vi "O to G v1.vi"(8 "height":dbl[](array[numeric]) format="%#_9g", 9 "south chip":dbl[](array[numeric]) format="%#_9g", 10 "north chip":dbl[](array[numeric]) format="%#_9g", 11 "Input file":path) -> (1 "output BR":dbl[](array[numeric]), 2 "output BL":dbl[](array[numeric]), 3 "output TL":dbl[](array[numeric]))   [LabVIEW 2016]
uses:
  <vilib>/Analysis/coordinate.llb/2D Cartesian Coordinate Rotation (Scalar).vi
  <vilib>/Utility/file.llb/Read Delimited Spreadsheet (DBL).vi
  <vilib>/Analysis/NI_AALPro.lvlib
panel:
  out "all rows":dbl[][](array[numeric])
  out "x+y":dbl[](array[numeric])
  out "Array":dbl[][](array[numeric]) format="%#_8g"
  out "south chip (1)":dbl[](array[numeric])
  out "north chip(2)":dbl[](array[numeric])
  out "south right (9)":dbl[](array[numeric])
  out "south left (10)":dbl[](array[numeric])
  out "north left(7)":dbl[](array[numeric])
  out "SC-NC":dbl[](array[numeric])
  out "rotation angle":dbl
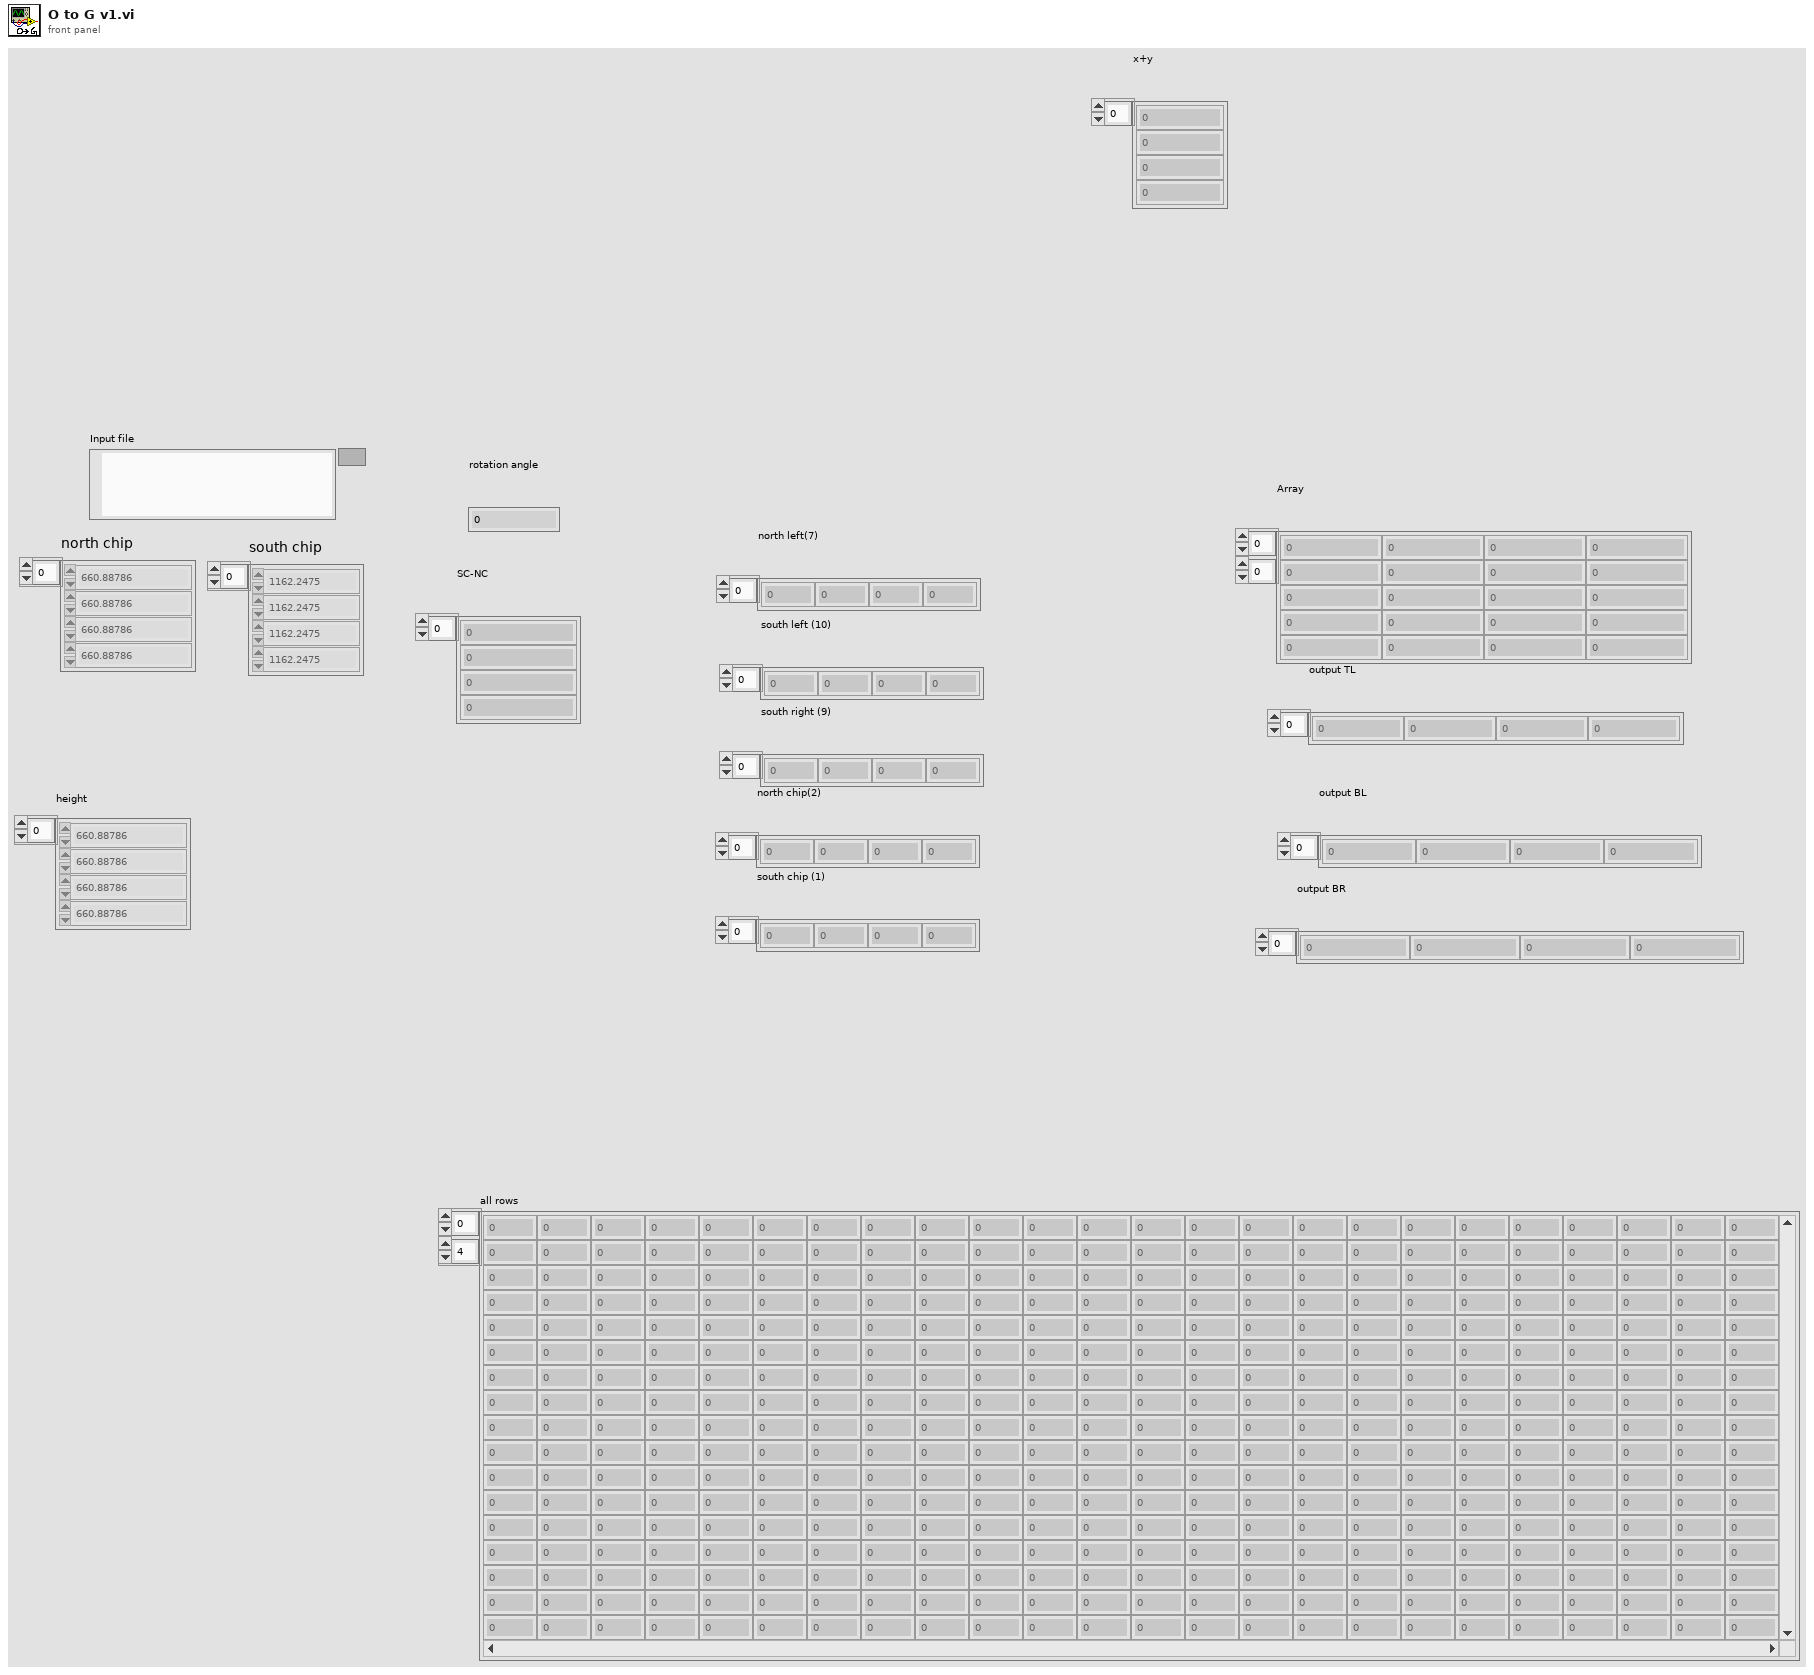
[diagram p1: front panel]
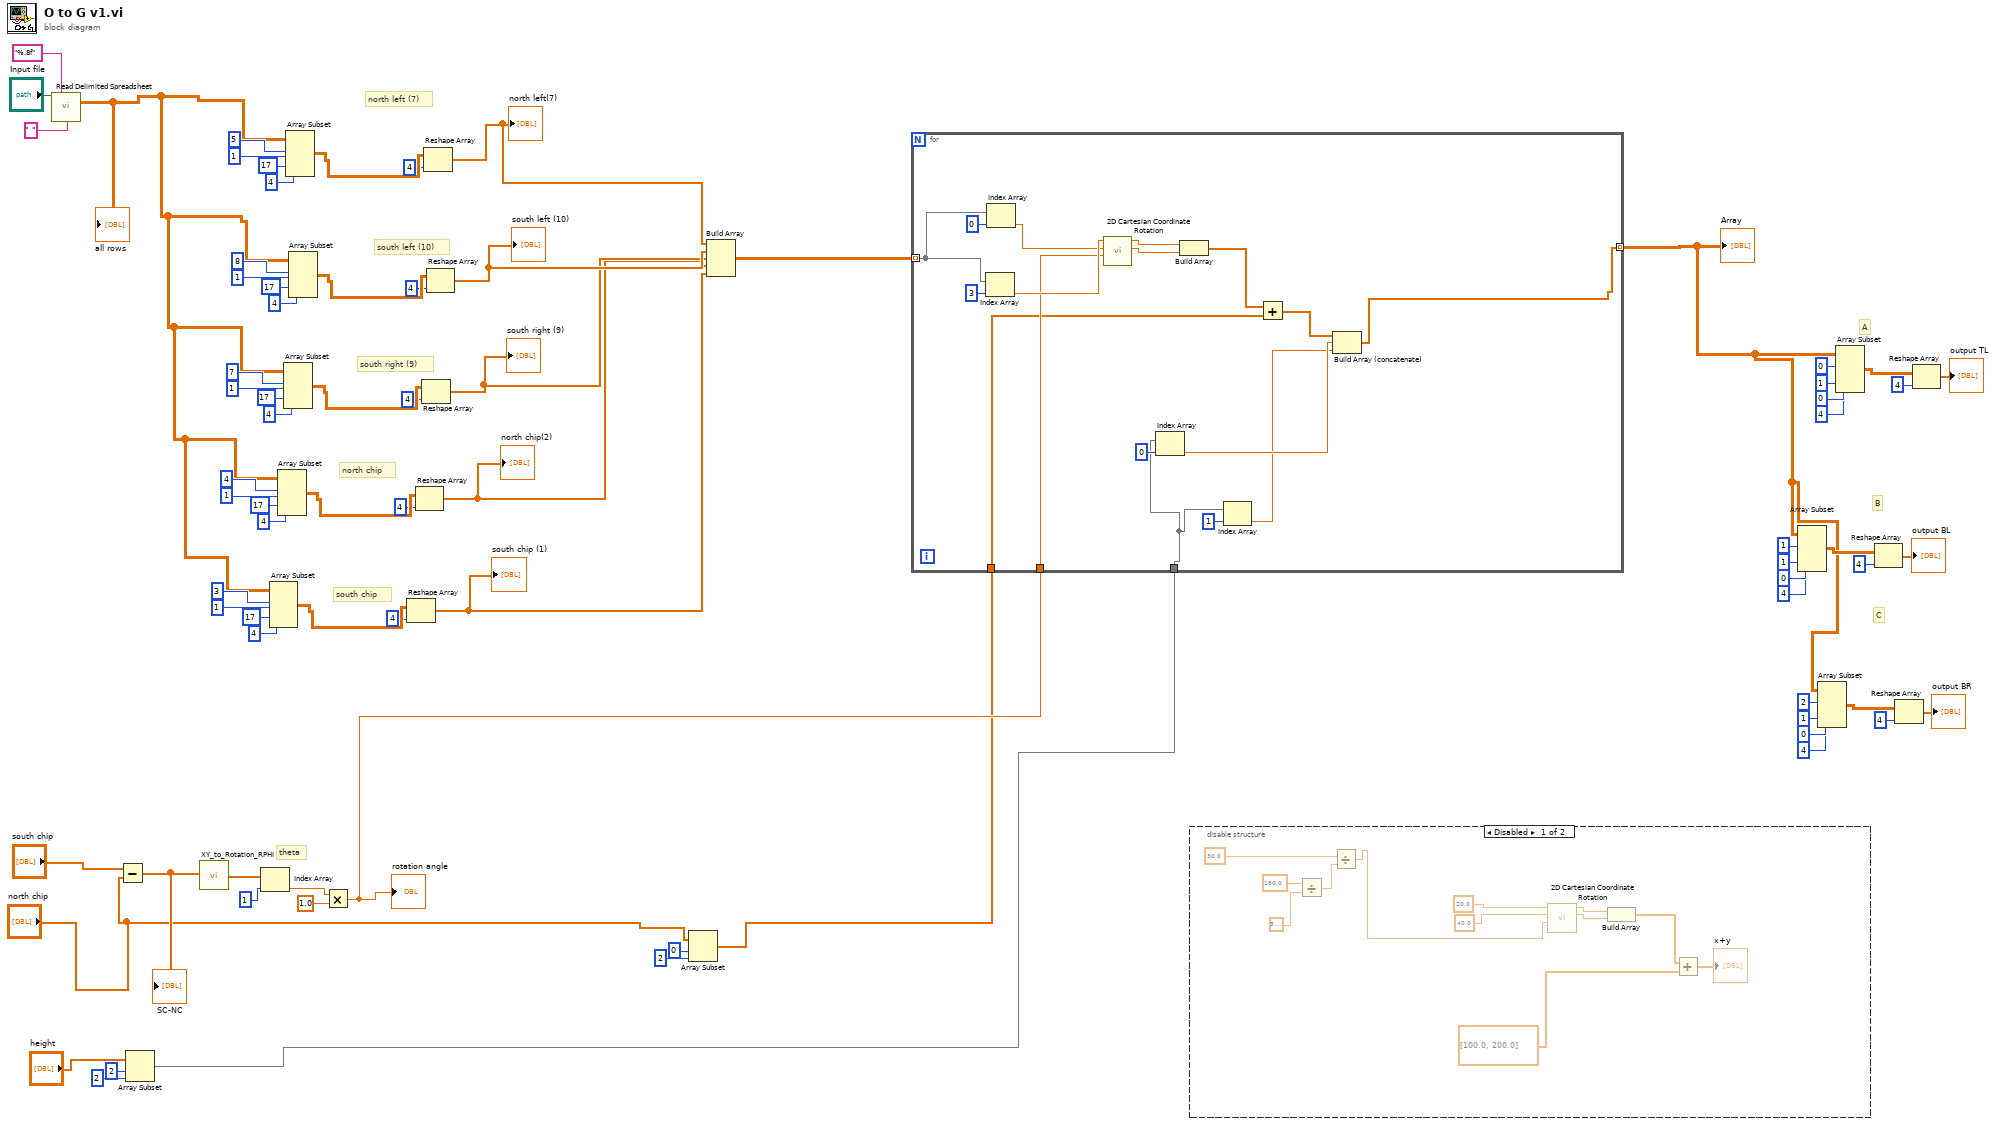
[diagram p0: block diagram]
diagram:
  # "C"
  # "B"
  # "A"
  # "south chip"
  # "north chip"
  # "south right (9)"
  # "south left (10)"
  # "north left (7)"
  # "theta"
  n1 = call-poly <vilib>:"Read Delimited Spreadsheet.vi"("file path (dialog if empty)"="Input file", "format (%.3f)"="%.8f", "delimiter (\\t)"=" " ("delimiter (\\t)")) -> ("all rows"=w40:dbl[][])  [unwired: 7 in, 5 out]
  "all rows" <- w40
  n2 = Subtract(x="south chip", y="north chip") -> (x-y=w71:dbl[])
  "SC-NC" <- w71
  n3 = Array Subset(array="height", index=2, length=2) -> (w27:dbl[])
  n4 = call "XY_to_Rotation_RPHI.vi"("X-Y"=w71) -> ("r-phi"=w74:dbl[])
  n5 = Index Array(array=w74, index=1) -> (element=w33:dbl)
  n6 = Array Subset(array=w40, index (row)=3 ("index"), length (row)=1 ("length"), index (col)=17 ("index"), length (col)=4 ("length")) -> (w42:dbl[][])
  n7 = Array Subset(array=w40, index (row)=4 ("index"), length (row)=1 ("length"), index (col)=17 ("index"), length (col)=4 ("length")) -> (w48:dbl[][])
  n8 = Array Subset(array=w40, index (row)=7 ("index"), length (row)=1 ("length"), index (col)=17 ("index"), length (col)=4 ("length")) -> (w54:dbl[][])
  n9 = Array Subset(array=w40, index (row)=5 ("index"), length (row)=1 ("length"), index (col)=17 ("index"), length (col)=4 ("length")) -> (w66:dbl[][])
  n10 = Array Subset(array=w40, index (row)=8 ("index"), length (row)=1 ("length"), index (col)=17 ("index"), length (col)=4 ("length")) -> (w60:dbl[][])
  n11 = Multiply(x=w33, y=1.0) -> (x*y=w32:dbl)
  "rotation angle" <- w32
  n12 = Reshape Array(w42, 4 ("dimension size")) -> (w35:dbl[])
  "south chip (1)" <- w35
  n13 = Reshape Array(w48, 4 ("dimension size")) -> (w36:dbl[])
  "north chip(2)" <- w36
  n14 = Reshape Array(w54, 4 ("dimension size")) -> (w37:dbl[])
  "south right (9)" <- w37
  n15 = Reshape Array(w66, 4 ("dimension size")) -> (w39:dbl[])
  "north left(7)" <- w39
  n16 = Reshape Array(w60, 4 ("dimension size")) -> (w38:dbl[])
  "south left (10)" <- w38
  n17 = Array Subset(array="north chip", index=0, length=2) -> (w23:dbl[])
  n18 = Build Array(w39, w38, w37, w36, w35) -> (w34:dbl[][])
  n19 = for {
    tunnel: w34 -> [w92] mode=indexing
    tunnel: w32 -> [w89]
    tunnel: [w78] -> w1 mode=indexing
    tunnel: w23 -> [w86]
    tunnel: w27 -> [w81]
    n20 = Index Array(array=w92, index=3) -> (element=w91:dbl)
    n21 = Index Array(array=w92, index=0) -> (element=w90:dbl)
    n22 = call-poly <vilib>:"2D Cartesian Coordinate Rotation.vi"("theta"=w89, "y"=w90, "x"=w91) -> ("y out"=w87:dbl, "x out"=w88:dbl)  [unwired: 6 in, 1 out]
    n23 = Index Array(array=w81, index=0) -> (element=w80:dbl)
    n24 = Build Array(w88, w87) -> (w85:dbl[])
    n25 = Index Array(array=w81, index=1) -> (element=w79:dbl)
    n26 = Add(x=w85, y=w86) -> (x+y=w84:dbl[])
    n27 = Build Array (concatenate)(w84, w80, w79) -> (w78:dbl[])
  }
  "Array" <- w1
  n28 = disable-structure shown="Disabled" {
    frame Disabled {
      n29 = Divide(x=180.0, y=3.141592653589793) -> (x/y=w103:dbl)
      n30 = Divide(x=30.0, y=w103) -> (x/y=w100:dbl)
      n31 = call-poly <vilib>:"2D Cartesian Coordinate Rotation.vi"("theta"=w100, "y"=40.0, "x"=20.0) -> ("y out"=w98:dbl, "x out"=w99:dbl)  [unwired: 6 in, 1 out]
      n32 = Build Array(w99, w98) -> (w97:dbl[])
      n33 = Add(x=w97, y=dbl[] [100.0, 200.0]) -> (x+y=→"x+y":dbl[])
    }
    frame Enabled {
    }
  }
  n34 = Array Subset(array=w1, index (row)=1 ("index"), length (row)=1 ("length"), index (col)=0 ("index"), length (col)=4 ("length")) -> (w15:dbl[][])
  n35 = Array Subset(array=w1, index (row)=2 ("index"), length (row)=1 ("length"), index (col)=0 ("index"), length (col)=4 ("length")) -> (w8:dbl[][])
  n36 = Array Subset(array=w1, index (row)=0 ("index"), length (row)=1 ("length"), index (col)=0 ("index"), length (col)=4 ("length")) -> (w22:dbl[][])
  n37 = Reshape Array(w15, 4 ("dimension size")) -> (→"output BL":dbl[])
  n38 = Reshape Array(w8, 4 ("dimension size")) -> (→"output BR":dbl[])
  n39 = Reshape Array(w22, 4 ("dimension size")) -> (→"output TL":dbl[])
